vi "tkrsa6100 Binary String Converter.vi"(9 "Digits of Precision\n(0)":i32 max=12 step=1, 10 "Binary Msmt Result String\n(Empty String)":string, 11 "Data Type\n(Sgl Float)":enum16{"Sgl Float", "32 Integer", "16 Integer"}(ring)) -> (1 "# Points":i32, 2 "Converted Result String":string)   [LabVIEW 2020, in "Library Instrument & Equipement.lvlib" / "Library Spectrum Analyser.lvlib"]
doc: "This VI converts the binary data string returned by some instrument queries to a comma separated string of single precision floating point numbers.\n\nIt functions as follows:\n\nSingle Float Return String is initialized to an empty string. The binary string response is passed to Binary Mmst Result String(Empty String).\n\nThe binary string format is #<num_digits><num_data_bytes><4 byte binary data>\n\nFirst <num_digits> is extracted by the String Subset function. It is one character at offset 1. It is converted to an uint32.\n\nNext <num_bytes> is extracted by the String Subset function. It starts at offset 2 and is <num_digits> long. It is converted to an uint32.\n\n<num_bytes> is divided by 4 to get the actual # of data points to convert (the binary data is 4 bytes/sample). The # of data points is then connected to the For Loop count terminal.\n\nThe binary string is fed to another String Subset function inside the while loop. This extracts 4 bytes from the string on each loop iteration. The index of the first sample is at <num_digits>+ 2 (# sign and <num_digits>). The 4 byte subset is passed to subvi Little Endian to Float.vi. This converts the string to a single precision floating point number. The float is converted to a string and appended onto Single Float Return String and a comma separator is added.\n\nOn the next loop iteration, the iteration terminal is at 1 instead of 0. This adds 4 to the starting offset value and the next 4 byte conversion proceeds. \n\nOn the last iteration, instead of adding a comma to Single Float Return String, it is terminated with an empty string. Single Float Return String is returned to the calling function."
uses:
  Library Spectrum Analyser.lvlib
panel:
  # "Convert Binary Result String to Sgl Precision Floats or 32 Bit Integers"
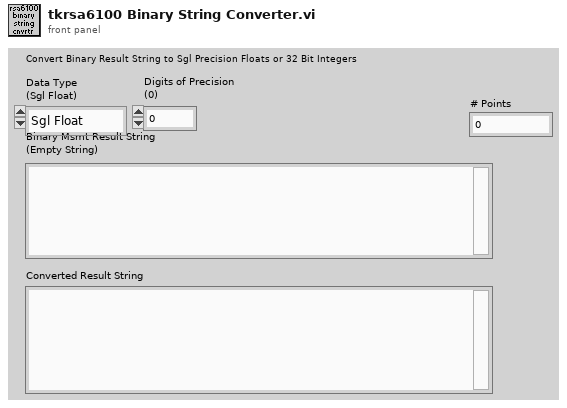
[diagram p1: front panel]
types:
  T1 = enum16{"big-endian, network order", "native, host order", "little-endian"}
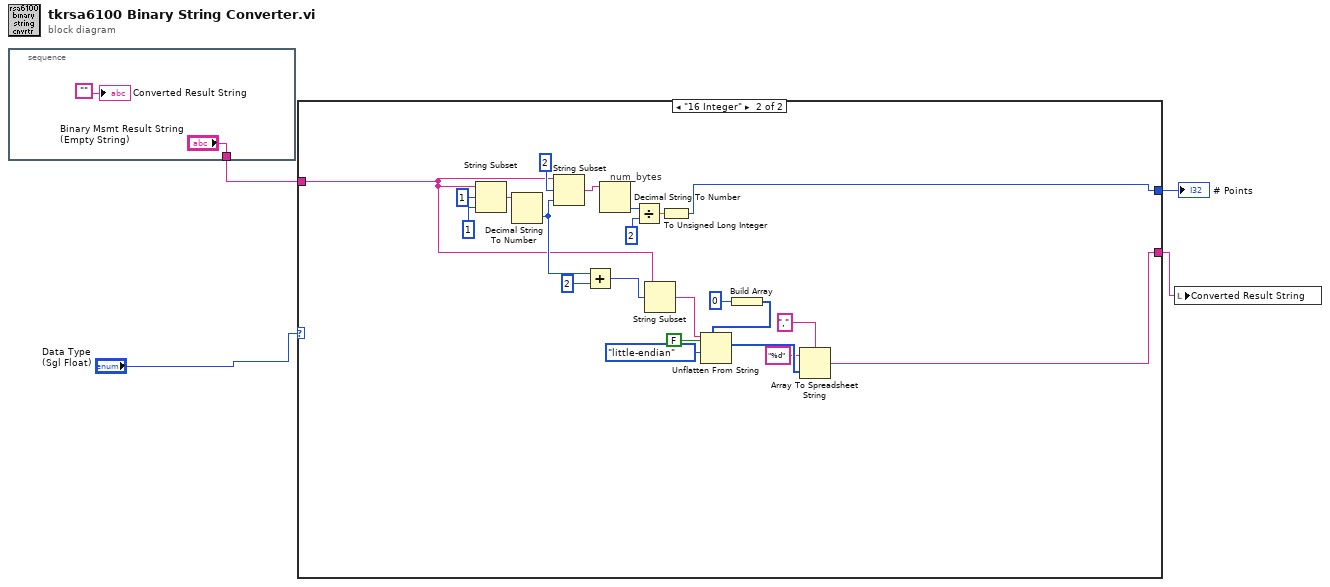
[diagram p0: block diagram]
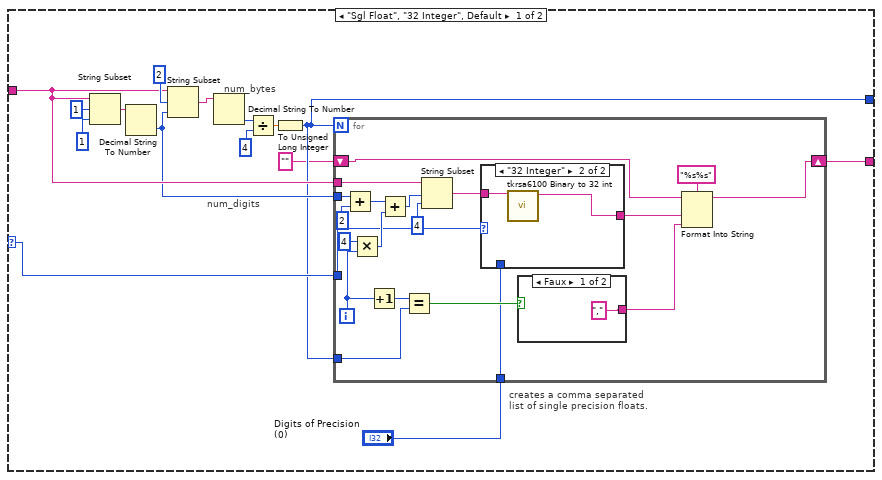
[diagram p2: hidden frame]
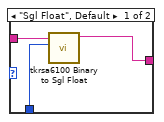
[diagram p3: hidden frame]
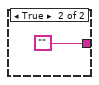
[diagram p4: hidden frame]
diagram:
  n1 = stacked-sequence {
    tunnel: ["Binary Msmt Result String\n(Empty String)"] -> w4
    frame #0 {
      "Converted Result String" <- ""
    }
  }
  n2 = case shown="\"16 Integer\"" "Data Type\n(Sgl Float)" {
    selector: "Data Type\n(Sgl Float)" -> [w10 _]
    tunnel: w4 -> [w14 w52]
    tunnel: [w9 w51] -> w2
    tunnel: [w7 w50] -> w1
    frame "Sgl Float", "32 Integer", Default {
      # "num_bytes"
      # "num_digits"
      # "creates a comma separated\nlist of single precision floats."
      n3 = String Subset(string=w14, offset (0)=1, length (rest)=1 ("length (rest)")) -> (substring=w18:string)
      n4 = Decimal String To Number(string=w18) -> (number=w12:i32)  [unwired: 3 out]
      n5 = String Subset(string=w14, offset (0)=2, length (rest)=w12) -> (substring=w17:string)
      n6 = Decimal String To Number(string=w17) -> (number=w13:i32)  [unwired: 3 out]
      n7 = Divide(x=w13, y=4) -> (x/y=w15:dbl)
      n8 = To Unsigned Long Integer(number=w15) -> (unsigned 32bit integer=w9:u32)
      n9 = for {
        N: w9 -> [_]
        tunnel: w14 -> [w41]
        tunnel: w12 -> [w35]
        tunnel: w9 -> [w31]
        tunnel: w10 -> [w25]
        tunnel: "Digits of Precision\n(0)" -> [w24]
        shift-right: [w22] -> w7
        shift-left: "" -> [w23]
        i -> [w33]
        n10 = Add(x=w35, y=u32 2) -> (x+y=w38:u32)
        n11 = Multiply(x=4, y=w33) -> (x*y=w37:i32)
        n12 = Increment(x=w33) -> (x+1=w32:i32)
        n13 = Add(x=w38, y=w37) -> (x+y=w36:u32)
        n14 = Equal?(x=w32, y=w31) -> (x = y?=w30:bool)
        n15 = String Subset(string=w41, offset (0)=w36, length (rest)=4 ("length (rest)")) -> (substring=w27:string)
        n16 = case shown="\"32 Integer\"" w25 {
          tunnel: w27 -> [w44 w46]
          tunnel: [w43 w45] -> w26
          tunnel: w24 -> [w42 _]
          frame "Sgl Float", Default {
            n17 = call "tkrsa6100 Binary to Sgl Float.vi"("Digits of Precision"=w42, "Character String"=w44) -> ("Float String"=w43:string)  [unwired: 9 out]
          }
          frame "32 Integer" {
            n18 = call "tkrsa6100 Binary to 32 int.vi"("Substring"=w46) -> ("String"=w45:string)  [unwired: 10 out]
          }
        }
        n19 = case shown="Faux" w30 {
          tunnel: ["," ("string") ""] -> w28
          frame False {
          }
          frame True {
          }
        }
        n20 = Format Into String(format string="%s%s", initial string=w23, w26, w28) -> (resulting string=w22:string)  [unwired: 1 in, 1 out]
      }
    }
    frame "16 Integer" {
      # "num_bytes"
      n21 = String Subset(string=w52, offset (0)=1, length (rest)=1 ("length (rest)")) -> (substring=w67:string)
      n22 = Decimal String To Number(string=w67) -> (number=w62:i32)  [unwired: 3 out]
      n23 = String Subset(string=w52, offset (0)=2, length (rest)=w62) -> (substring=w66:string)
      n24 = Add(x=w62, y=2) -> (x+y=w53:i32)
      n25 = Decimal String To Number(string=w66) -> (number=w63:i32)  [unwired: 3 out]
      n26 = Divide(x=w63, y=2) -> (x/y=w64:dbl)
      n27 = String Subset(string=w52, offset (0)=w53) -> (substring=w60:string)  [unwired: 1 in]
      n28 = To Unsigned Long Integer(number=w64) -> (unsigned 32bit integer=w51:u32)
      n29 = Build Array(u16 0) -> (w57:u16[])
      n30 = Unflatten From String(type=w57, binary string=w60, data includes array or string size? (T)=FALSE, byte order (0:big-endian, network order)=T1."little-endian") -> (value=w56:u16[])  [unwired: 1 in, 2 out]
      n31 = Array To Spreadsheet String(delimiter (Tab)=",", array=w56, 3:"%d" ("format string")) -> (spreadsheet string=w50:string)
    }
  }
  "# Points" <- w2
  n32 = local write "Converted Result String"(w1) -> ()
